vi "is_empty.vi"(8 "error in (no error)":errorcluster, 11 "DoublyLinkedList in":refnum<class "DoublyLinkedList.lvclass">) -> (0 "error out":errorcluster, 1 "empty?":bool, 3 "DoublyLinkedList out":refnum<class "DoublyLinkedList.lvclass">)   [LabVIEW 2021, in "DoublyLinkedList.lvclass"]
uses:
  DoublyLinkedList.lvclass
  DoublyLinkedList.lvclass/DoublyLinkedList.ctl
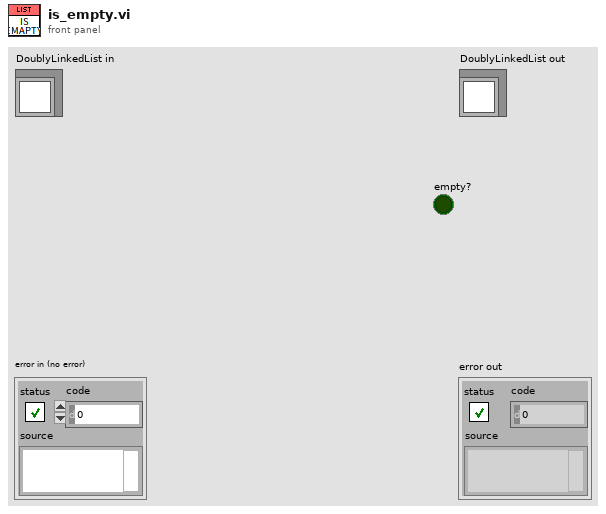
[diagram p1: front panel]
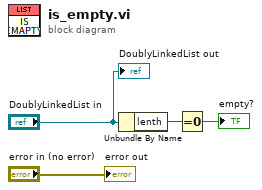
[diagram p0: block diagram]
diagram:
  n1 = Unbundle By Name("DoublyLinkedList in") -> ("lenth"=w2:u32)
  n2 = Equal To 0?(x=w2) -> (x = 0?=→"empty?":bool)
  "error out" <- "error in (no error)"
  "DoublyLinkedList out" <- "DoublyLinkedList in"
